vi "generate task plan.vi"() -> (1 "stage plan":T6[][](array[typedef]), 3 "do waveforms":T4[](array[typedef]))   [LabVIEW 2015]
uses:
  type def/stage plan.ctl
  type def/task plan.ctl
  type def/do waveform.ctl
  type def/task status.ctl
  type def/basic params.ctl
  type def/advanced params.ctl
  global variables/params.vi
panel:
  in  "advanced params":T1={"x flyback time(%)"=40.0, "signal offset"=0, "frame time(s)"=0.0, "fetch # per frame"=1, "galvo sampling rate"=500000} {"galvo sampling rate" min=10000 max=200000 step=1; "fetch # per frame" min=1 max=100 step=1 format="%#.3g"; "frame time(s)" min=0.0 max=100.0 step=0.1 format="%#.3g"; "signal offset" max=10000 format="%#.3g"; "x flyback time(%)" min=0.0 max=50.0 format="%#.3g"}
  in  "basic params":T2={"X pixel #"=200, "X pixel size(um)"=1.0, "Y pixel #"=200, "Y pixel size(um)"=10.0, "line rate(Hz)"=1.0, "stage scan?"=FALSE} {"line rate(Hz)" min=1.0 max=2000.0 format="%#.3g"; "X pixel size(um)" min=0.0 max=10.0 format="%#.3g"; "X pixel #" min=2 max=20480 step=2 format="%#.3g"; "Y pixel size(um)" min=0.0 max=10.0 format="%#.3g"; "Y pixel #" min=2 max=204800 step=2 format="%#.3g"}
  out "task status":T3
  in  "task plan":T5 {"Z end" min=0.0; "Z start" min=0.0; "Y end" min=0.0; "Y start" min=0.0; "X overlap" min=0.0; "X end" min=0.0; "X start" min=0.0}
  # "write"
  # "scan"
  # "in"
  # "z block"
  # "in"
  # "x block"
  # "in"
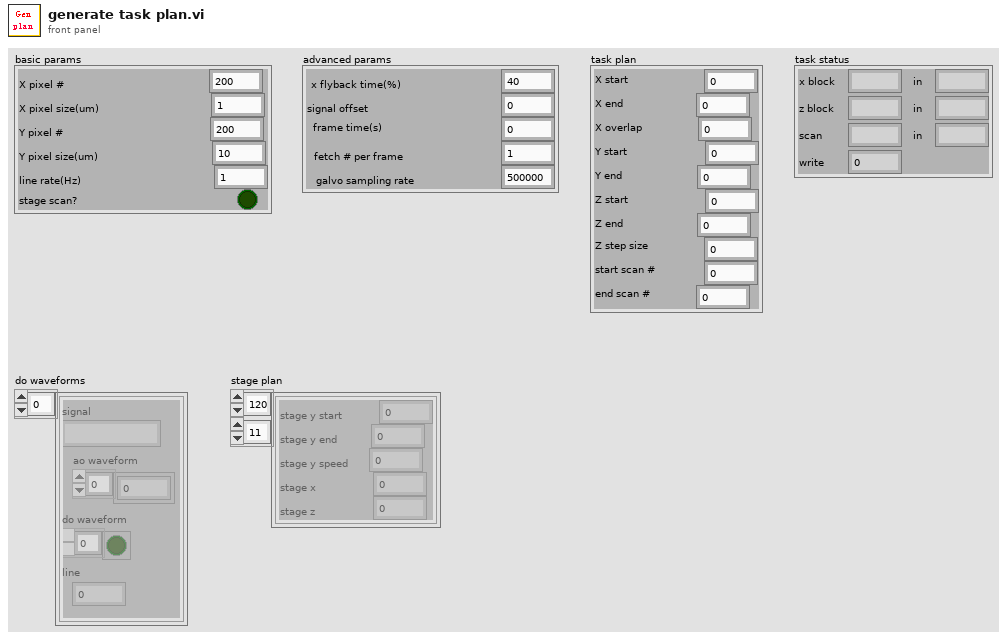
[diagram p1: front panel]
types:
  T1 = typedef "advanced params.ctl" = cluster{"x flyback time(%)":dbl, "signal offset":u16, "frame time(s)":dbl, "fetch # per frame":u16, "galvo sampling rate":u32}
  T2 = typedef "basic params.ctl" = cluster{"X pixel #":u32, "X pixel size(um)":dbl, "Y pixel #":u32, "Y pixel size(um)":dbl, "line rate(Hz)":dbl, "stage scan?":bool}
  T3 = typedef "task status.ctl" = cluster{"xn":u16, "x total":u16, "zn":u16, "z total":u16, "scan n":u16, "scan total":u16, "write":u16}
  T4 = typedef "do waveform.ctl" = cluster{"signal":string, "ao waveform":dbl[], "do waveform":bool[], "line":u8}
  T5 = typedef "task plan.ctl" = cluster{"X start":dbl, "X end":dbl, "X overlap":dbl, "Y start":dbl, "Y end":dbl, "Z start":dbl, "Z end":dbl, "Z step size":dbl, "start scan #":u16, "end scan #":u16}
  T6 = typedef "stage plan.ctl" = cluster{"stage y start":dbl, "stage y end":dbl, "stage y speed":dbl, "stage x":dbl, "stage z":dbl}
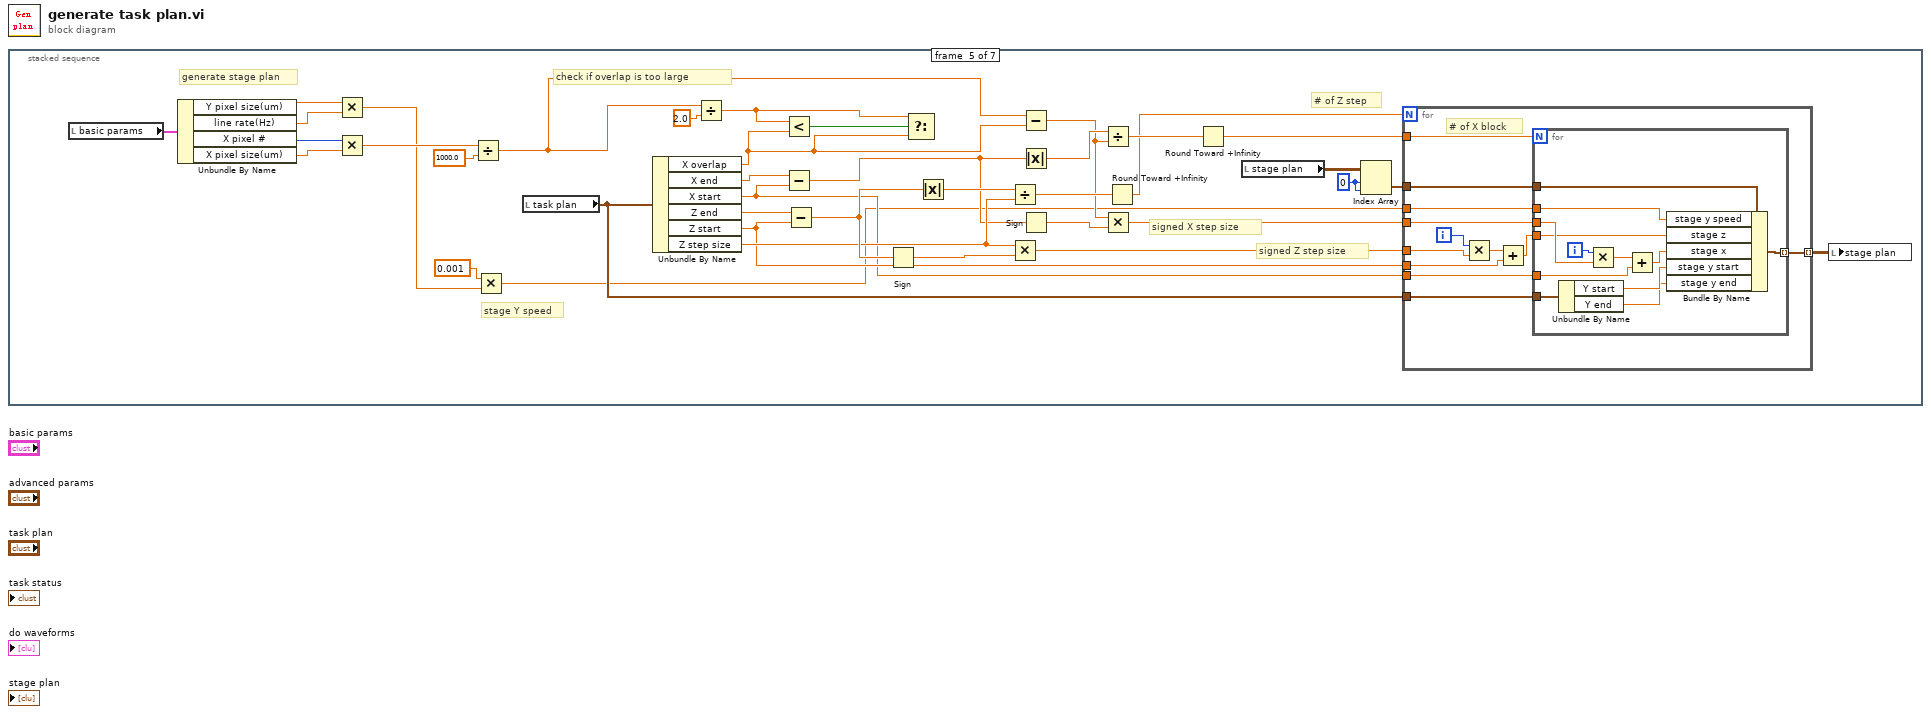
[diagram p0: block diagram]
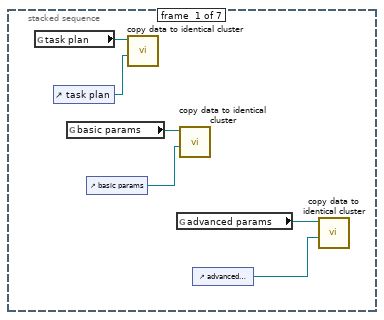
[diagram p2: hidden frame]
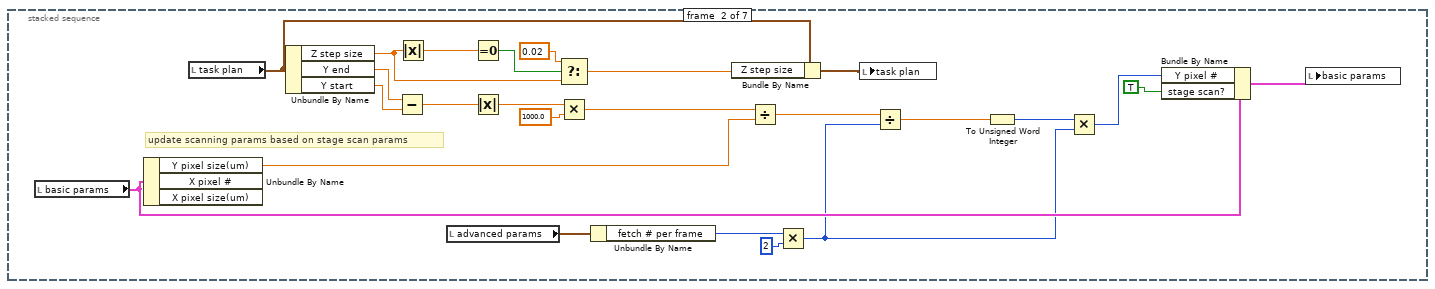
[diagram p3: hidden frame]
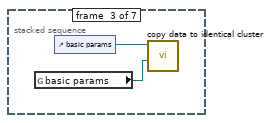
[diagram p4: hidden frame]
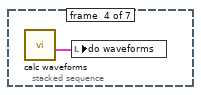
[diagram p5: hidden frame]
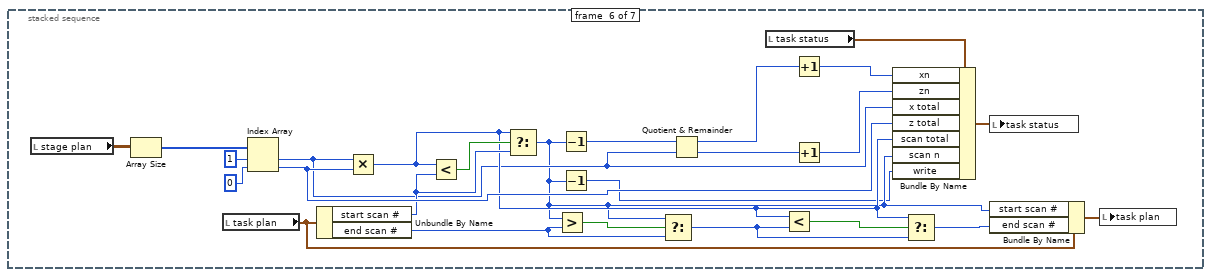
[diagram p6: hidden frame]
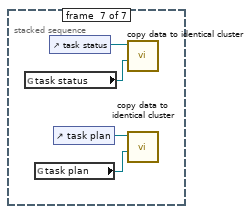
[diagram p7: hidden frame]
diagram:
  n1 = stacked-sequence {
    frame #0 {
      n2 = global read "params.vi" "task plan"() -> (w3:refnum<vi>)
      n3 = control-ref of="task plan"() -> (w4:refnum<vi>)
      n4 = global read "params.vi" "basic params"() -> (w6:refnum<vi>)
      n5 = control-ref of="basic params"() -> (w2:refnum<vi>)
      n6 = call "copy data to identical cluster.vi"("Guest Clust Refnum"=w4, "Host Clust Refnum"=w3) -> ()  [unwired: 10 in]
      n7 = global read "params.vi" "advanced params"() -> (w5:refnum<vi>)
      n8 = call "copy data to identical cluster.vi"("Guest Clust Refnum"=w2, "Host Clust Refnum"=w6) -> ()  [unwired: 10 in]
      n9 = control-ref of="advanced params"() -> (w1:refnum<vi>)
      n10 = call "copy data to identical cluster.vi"("Guest Clust Refnum"=w1, "Host Clust Refnum"=w5) -> ()  [unwired: 10 in]
    }
    frame #1 {
      # "update scanning params based on stage scan params"
      n11 = local read "basic params"() -> (w31:T2)
      n12 = Unbundle By Name(w31) -> ("Y pixel size(um)"=w7:dbl)  [unwired: 2 out]
      n13 = local read "task plan"() -> (w10:T5)
      n14 = Unbundle By Name(w10) -> ("Z step size"=w12:dbl, "Y end"=w28:dbl, "Y start"=w29:dbl)
      n15 = Subtract(x=w28, y=w29) -> (x-y=w27:dbl)
      n16 = Absolute Value(x=w12) -> (abs(x)=w14:dbl)
      n17 = local read "advanced params"() -> (w30:T1)
      n18 = Equal To 0?(x=w14) -> (x = 0?=w13:bool)
      n19 = Absolute Value(x=w27) -> (abs(x)=w23:dbl)
      n20 = Select(t=0.02, s=w13, f=w12) -> (s? t:f=w9:dbl)
      n21 = Multiply(x=w23, y=1000.0) -> (x*y=w22:dbl)
      n22 = Unbundle By Name(w30) -> ("fetch # per frame"=w26:u16)
      n23 = Bundle By Name(cluster=w10, "Z step size"=w9) -> (w8:T5)
      n24 = Divide(x=w22, y=w7) -> (x/y=w21:dbl)
      n25 = Multiply(x=w26, y=u8 2) -> (x*y=w18:u16)
      n26 = local write "task plan"(w8) -> ()
      n27 = Divide(x=w21, y=w18) -> (x/y=w20:dbl)
      n28 = To Unsigned Word Integer(number=w20) -> (unsigned 16bit integer=w19:u16)
      n29 = Multiply(x=w19, y=w18) -> (x*y=w17:u16)
      n30 = Bundle By Name(cluster=w31, "Y pixel #"=w17, "stage scan?"=TRUE) -> (w15:T2)
      n31 = local write "basic params"(w15) -> ()
    }
    frame #2 {
      n32 = global read "params.vi" "basic params"() -> (w33:refnum<vi>)
      n33 = control-ref of="basic params"() -> (w32:refnum<vi>)
      n34 = call "copy data to identical cluster.vi"("Guest Clust Refnum"=w33, "Host Clust Refnum"=w32) -> ()  [unwired: 10 in]
    }
    frame #3 {
      n35 = call "calc waveforms.vi"() -> ("do waveforms"=w34:T4[])  [unwired: 10 in]
      n36 = local write "do waveforms"(w34) -> ()
    }
    frame #4 {
      w38 = 0 ("disabled index (col)")
      # "stage Y speed"
      # "generate stage plan"
      # "signed X step size"
      # "signed Z step size"
      # "# of Z step"
      # "check if overlap is too large"
      n37 = local read "basic params"() -> (w72:T2)
      n38 = Unbundle By Name(w72) -> ("Y pixel size(um)"=w42:dbl, "line rate(Hz)"=w43:dbl, "X pixel #"=w71:u32, "X pixel size(um)"=w70:dbl)
      n39 = Multiply(x=w42, y=w43) -> (x*y=w41:dbl)
      n40 = Multiply(x=w71, y=w70) -> (x*y=w69:dbl)
      n41 = Divide(x=w69, y=1000.0) -> (x/y=w64:dbl)
      n42 = Multiply(x=0.001, y=w41) -> (x*y=w39:dbl)
      n43 = local read "task plan"() -> (w45:T5)
      n44 = Unbundle By Name(w45) -> ("X overlap"=w35:dbl, "X end"=w63:dbl, "X start"=w47:dbl, "Z end"=w60:dbl, "Z start"=w51:dbl, "Z step size"=w55:dbl)
      n45 = Divide(x=w64, y=2.0) -> (x/y=w65:dbl)
      n46 = Less?(x=w65, y=w35) -> (x < y?=w66:bool)
      n47 = Subtract(x=w63, y=w47) -> (x-y=w50:dbl)
      n48 = Subtract(x=w60, y=w51) -> (x-y=w57:dbl)
      n49 = Sign(1:w57) -> (0:w56:dbl)
      n50 = Select(t=w65, s=w66, f=w35) -> ()  [unwired: 1 out]
      n51 = Absolute Value(x=w57) -> (abs(x)=w59:dbl)
      n52 = Divide(x=w59, y=w55) -> (x/y=w58:dbl)
      n53 = Multiply(x=w55, y=w56) -> (x*y=w54:dbl)
      n54 = Subtract(x=w64, y=w35) -> (x-y=w49:dbl)
      n55 = Absolute Value(x=w50) -> (abs(x)=w62:dbl)
      n56 = Sign(1:w50) -> (0:w48:dbl)
      n57 = Divide(x=w62, y=w49) -> (x/y=w61:dbl)
      n58 = Multiply(x=w49, y=w48) -> (x*y=w46:dbl)
      n59 = Round Toward +Infinity(x=w58) -> (ceil(x): smallest int >= x=w37:dbl)
      n60 = Round Toward +Infinity(x=w61) -> (ceil(x): smallest int >= x=w36:dbl)
      n61 = local read "stage plan"() -> (w53:T6[][])
      n62 = Index Array(array=w53, index (row)=w38, index (col)=w38) -> (element=w52:T6)
      n63 = for {
        N: w37 -> [_]
        tunnel: w36 -> [w84]
        tunnel: w54 -> [w73]
        tunnel: w52 -> [w83]
        tunnel: w51 -> [w77]
        tunnel: w47 -> [w75]
        tunnel: w46 -> [w78]
        tunnel: w45 -> [w81]
        tunnel: [w80] -> w44 mode=indexing
        tunnel: w39 -> [w79]
        i -> [w74]
        # "# of X block"
        n64 = Multiply(x=w74, y=w73) -> (x*y=w76:dbl)
        n65 = Add(x=w76, y=w77) -> (x+y=w82:dbl)
        n66 = for {
          N: w84 -> [_]
          tunnel: w83 -> [w96]
          tunnel: w78 -> [w92]
          tunnel: w75 -> [w94]
          tunnel: w82 -> [w90]
          tunnel: w81 -> [w89]
          tunnel: [w86] -> w80 mode=indexing
          tunnel: w79 -> [w85]
          i -> [w93]
          n67 = Unbundle By Name(w89) -> ("Y start"=w88:dbl, "Y end"=w87:dbl)
          n68 = Multiply(x=w93, y=w92) -> (x*y=w91:dbl)
          n69 = Add(x=w91, y=w94) -> (x+y=w95:dbl)
          n70 = Bundle By Name(cluster=w96, "stage y speed"=w85, "stage z"=w90, "stage x"=w95, "stage y start"=w88, "stage y end"=w87) -> (w86:T6)
        }
      }
      n71 = local write "stage plan"(w44) -> ()
    }
    frame #5 {
      n72 = local read "stage plan"() -> (w121:T6[][])
      n73 = Array Size(array=w121) -> (size(s)=w120:i32[])
      n74 = local read "task plan"() -> (w107:T5)
      n75 = Index Array(array=w120, index #1=1 ("index"), index #2=0 ("index")) -> (element #1=w104:i32, element #2=w116:i32)
      n76 = Unbundle By Name(w107) -> ("start scan #"=w113:u16, "end scan #"=w111:u16)
      n77 = Multiply(x=w104, y=w116) -> (x*y=w109:i32)
      n78 = Less?(x=w109, y=w113) -> (x < y?=w114:bool)
      n79 = Select(t=w109, s=w114, f=w113) -> (s? t:f=w98:i32)
      n80 = Greater?(x=w98, y=w111) -> (0:w112:bool)
      n81 = Decrement(x=w98) -> (x-1=w103:i32)
      n82 = Decrement(x=w98) -> (x-1=w97:i32)
      n83 = Select(t=w98, s=w112, f=w111) -> (s? t:f=w108:i32)
      n84 = Quotient & Remainder(x=w103, y=w104) -> (x-y*floor(x/y)=w100:i32, floor(x/y)=w102:i32)
      n85 = local read "task status"() -> (w117:T3)
      n86 = Less?(x=w109, y=w108) -> (x < y?=w110:bool)
      n87 = Increment(x=w100) -> (x+1=w99:i32)
      n88 = Increment(x=w102) -> (x+1=w101:i32)
      n89 = Bundle By Name(cluster=w117, "xn"=w99, "zn"=w101, "x total"=w104, "z total"=w116, "scan total"=w109, "scan n"=w98, "write"=w97) -> (w115:T3)
      n90 = Select(t=w109, s=w110, f=w108) -> (s? t:f=w106:i32)
      n91 = local write "task status"(w115) -> ()
      n92 = Bundle By Name(cluster=w107, "start scan #"=w98, "end scan #"=w106) -> (w105:T5)
      n93 = local write "task plan"(w105) -> ()
    }
    frame #6 {
      n94 = global read "params.vi" "task status"() -> (w125:refnum<vi>)
      n95 = global read "params.vi" "task plan"() -> (w123:refnum<vi>)
      n96 = control-ref of="task status"() -> (w124:refnum<vi>)
      n97 = control-ref of="task plan"() -> (w122:refnum<vi>)
      n98 = call "copy data to identical cluster.vi"("Guest Clust Refnum"=w125, "Host Clust Refnum"=w124) -> ()  [unwired: 10 in]
      n99 = call "copy data to identical cluster.vi"("Guest Clust Refnum"=w123, "Host Clust Refnum"=w122) -> ()  [unwired: 10 in]
    }
  }
